vi "GetNodeMenuOption.vi"(0 "reference":refnum<class "ClassRelationshipEdge.lvclass">, 5 "error in (no error)":errorcluster) -> (14 "reference out":refnum<class "ClassRelationshipEdge.lvclass">, 15 "MenuOptions":string[](array[string]), 19 "error out":errorcluster)   [LabVIEW 2014, in "ClassRelationshipEdge.lvclass"]
doc: "Get Menu option"
uses:
  <resource>/Framework/Providers/Open_GDS/UML/ClassRelationshipEdge_class/ClassRelationshipEdge.lvclass
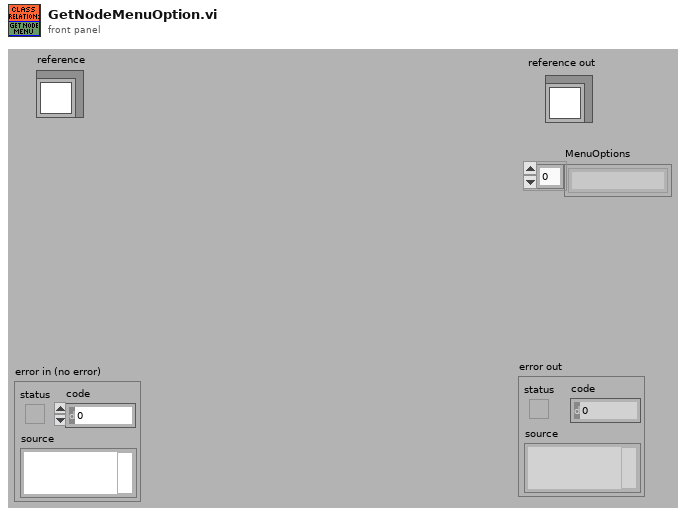
[diagram p1: front panel]
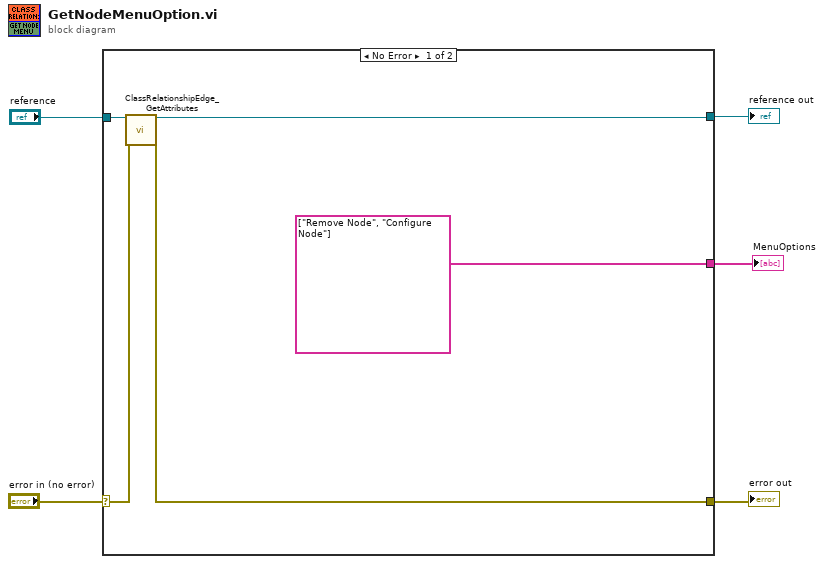
[diagram p0: block diagram]
diagram:
  n1 = case shown="No Error" "error in (no error)" {
    selector: "error in (no error)" -> [w10 w11]
    tunnel: "reference" -> [w9 w12]
    tunnel: [w7 w11] -> w3
    tunnel: [w8 w12] -> w2
    tunnel: [string[] ["Remove Node", "Configure Node"] _] -> w1
    frame No Error {
      n2 = call <resource>:"ClassRelationshipEdge_GetAttributes.vi"("reference in"=w9, "error in (no error)"=w10) -> ("reference out"=w8:refnum<class "ClassRelationshipEdge.lvclass">, "error out"=w7:errorcluster)  [unwired: 1 in, 15 out]
    }
    frame Error {
    }
  }
  "reference out" <- w2
  "error out" <- w3
  "MenuOptions" <- w1
